vi "AM-Amplitude Modulation-Sound Output.vi"() -> ()   [LabVIEW 2016]
uses:
  <vilib>/sound2/lvsound2.llb/Sound Data Format.ctl
  <vilib>/Platform/TimedLoop/XDataNode/timing_clust.ctl
  <vilib>/Platform/TimedLoop/XDataNode/nitl_modes.ctl
  <vilib>/Platform/TimedLoop/XDataNode/wakeup.ctl
  <vilib>/measure/maspectr.llb/FFT Power Spectrum for 1 Chan.vi
  <vilib>/sound2/lvsound2.llb/Sound Output Write (DBL Single).vi
  <vilib>/Platform/TimedLoop/XDataNode/XDataNode.xnode
  <vilib>/Analysis/NI_AALBase.lvlib
  <vilib>/measure/NI_MAPro.lvlib
  <vilib>/Platform/TimedLoop/XDataNode/XDNodeRunTimeDep.lvlib
panel:
  in  "device ID":u32
  out "Data Signal":waveform(dbl)(graph) caption="Data Wave (Time Domain)"
  out "AM Modulated Signal (Frequency Domain)":cluster{"f0":dbl, "df":dbl, "magnitude":dbl[]}(graph) caption="AM Wave in Frequency Domain"
  out "Carrier Signal":waveform(dbl)(graph) caption="Carrier Wave (Time Domain)"
  out "AM Modulated Signal (Time Domain)":waveform(dbl)(graph) caption="AM Wave in Time Domain"
  in  "Carrier Amplitude":dbl(slide)=0.5 caption="Amplitude" min=0.0 max=1.0 scale=0.0..1.0
  in  "Data Frequency":dbl(slide)=40.0 caption="Frequency" scale=0.0..200.0
  in  "stop":bool
  in  "Data Amplitude":dbl(slide)=0.5 caption="Amplitude" min=0.0 max=1.0 scale=0.0..1.0
  in  "Carrier Frequency":dbl(slide)=400.0 caption="Frequency" scale=0.0..2000.0
  # "AM - Amplitude Modulation"
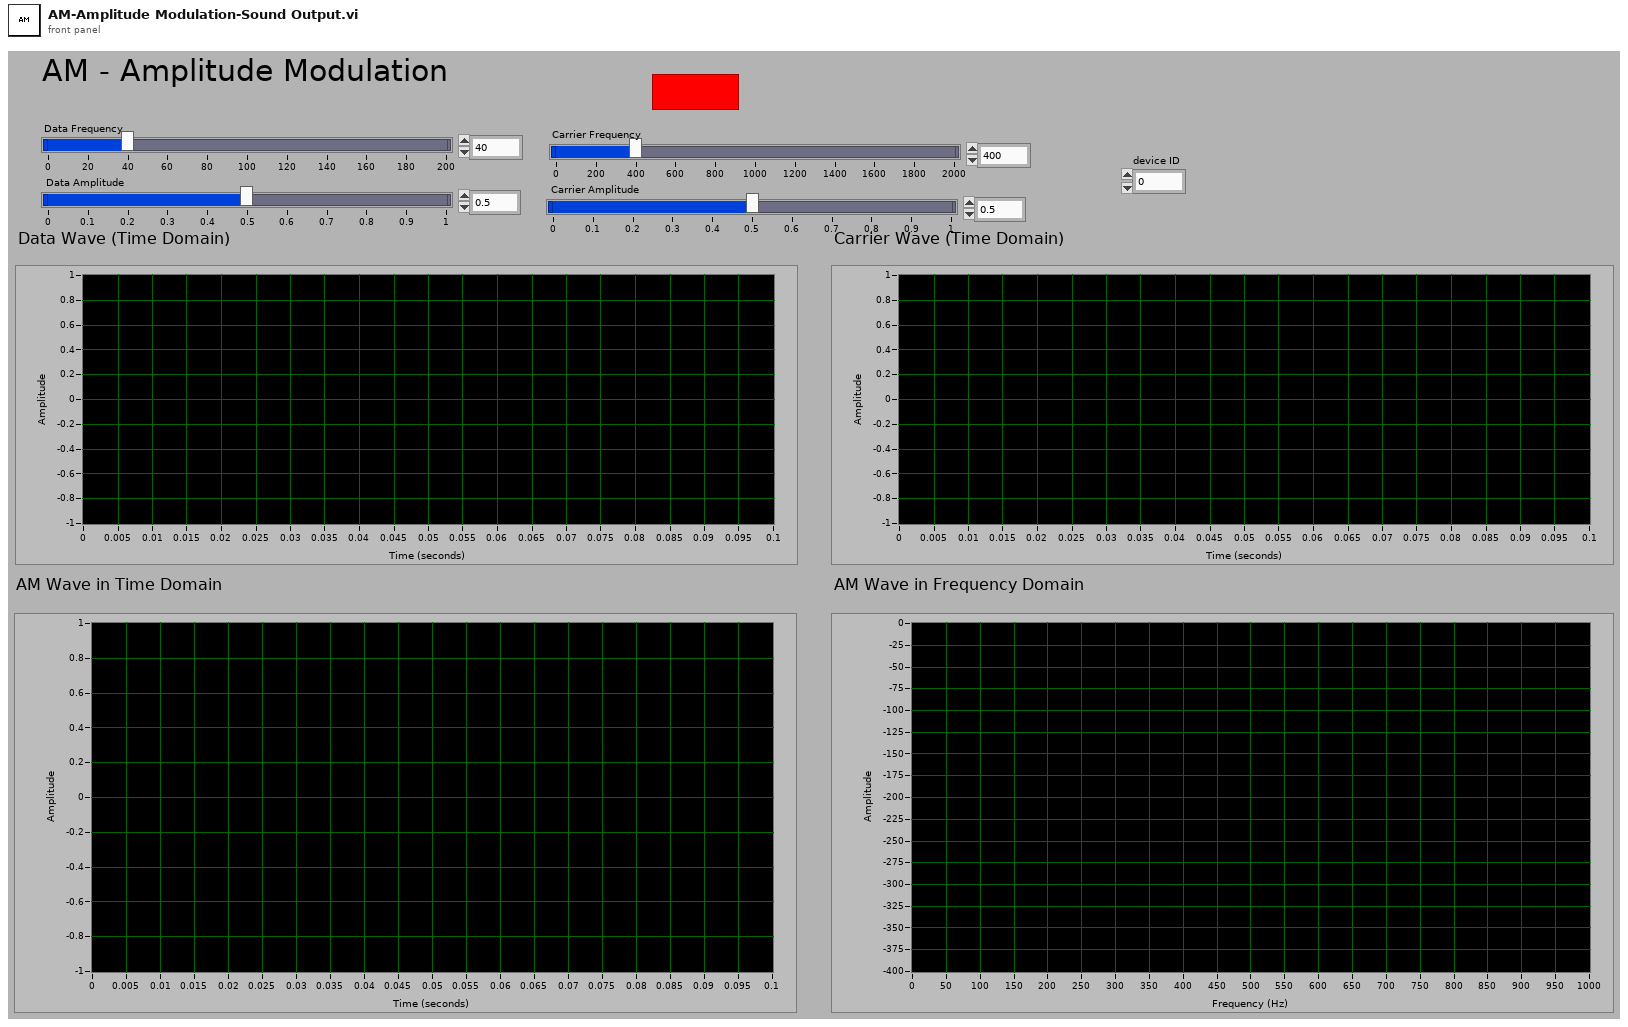
[diagram p1: front panel]
types:
  T1 = typedef "Sound Data Format.ctl" = cluster{"sample rate (S/s)":dbl, "number of channels":i32, "bits per sample":i32}
  T2 = typedef "Sound Output Task ID.ctl" = u32
  T3 = typedef "XDNodeRunTimeDep.lvlib/timing_clust.ctl" = cluster{"Expected End [f-1]":u64, "Actual End [f-1]":u64, "Finished Late? [f-1]":bool, "Expected End [i-1]":u64, "Actual End [i-1]":u64, "Finished Late? [i-1]":bool, "Expected Start [i]":u64, "Actual Start [i]":u64, "Expected Start [f]":u64, "Actual Start [f]":u64, "Source Name":string, "Structure Name":string, "Period":i64, "Deadline":i64, "Offset":i64, "Start":i64, "Priority":i32, "Timeout":i32, "Mode":T4, "Wakeup Reason":T5, "Error":errorcluster, "Source Type":string, "Secondary Source Type":string, "Global End Time":u64, "Global Start Time":u64, "Frame Duration":u64, "Iteration Duration":u64, "Assigned CPU":i32, "I/O Scan Engine Mode":u32}
  T4 = typedef "XDNodeRunTimeDep.lvlib/nitl_modes.ctl" = enum32{"No Change", "Process missed periods, maintain original phase", "Discard missed periods, maintain original phase", "Process missed periods, ignore original phase", "Discard missed periods, ignore original phase"}
  T5 = typedef "XDNodeRunTimeDep.lvlib/wakeup.ctl" = enum32{"Normal", "Aborted", "Asynchronous wakeup", "Timing source error", "Timed loop error", "Timeout"}
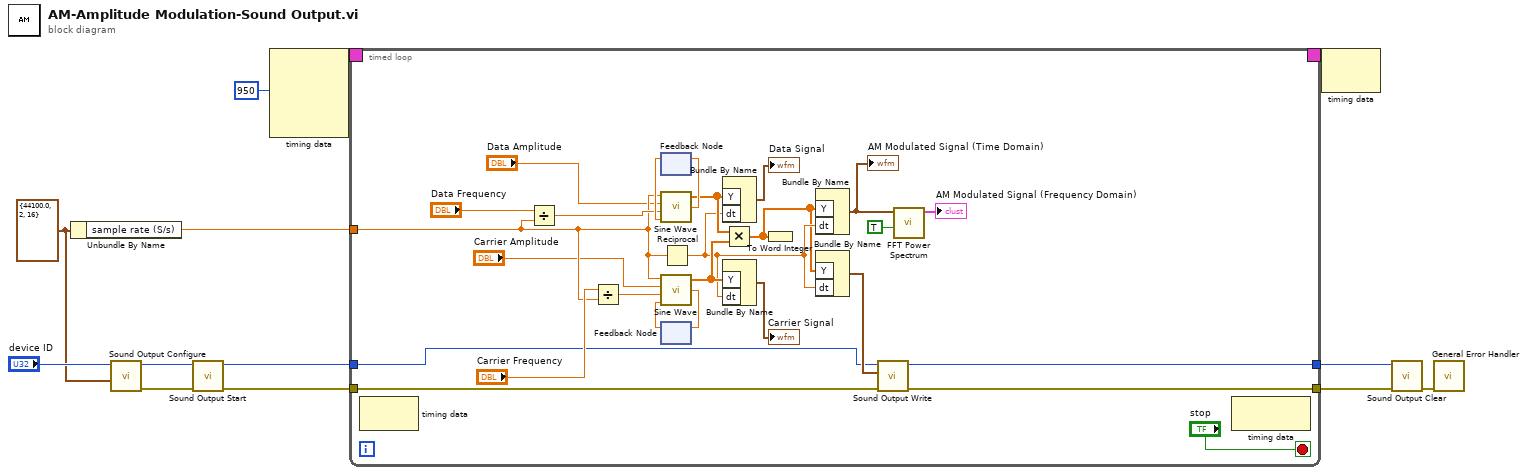
[diagram p0: block diagram]
diagram:
  w5 = T1 {"sample rate (S/s)"=44100.0, "number of channels"=2, "bits per sample"=16} ("sound format")
  n1 = Unbundle By Name(w5) -> ("sample rate (S/s)"=w4:dbl)
  n2 = call <vilib>:"Sound Output Configure.vi"("sound format"=w5, "device ID"="device ID") -> ("error out"=w11:errorcluster, "task ID"=w12:T2)  [unwired: 8 in]
  n3 = call <vilib>:"Sound Output Start.vi"("error in (no error)"=w11, "task ID"=w12) -> ("error out"=w9:errorcluster, "task ID out"=w10:T2)  [unwired: 8 in]
  n4 = node-c288(i64 950 ("Period")) -> (w3:T3)  [unwired: 3 in]
  n5 = timed-loop {
    tunnel: w10 -> [w18]
    tunnel: w9 -> [w17]
    tunnel: [w21] -> w8
    tunnel: [w20] -> w7
    tunnel: w4 -> [w30]
    timing: w3 -> [_]
    timing-out: [_] -> w2
    stop <- "stop" stop-if-true
    n6 = node-c288() -> ()  [unwired: 1 in, 1 out]
    n7 = Divide(x="Data Frequency", y=w30) -> (x/y=w35:dbl)
    n8 = Divide(x="Carrier Frequency", y=w30) -> (x/y=w31:dbl)
    n9 = feedback #1() -> (w37:dbl)  [unwired: 1 in]
    n10 = call <vilib>:"Sine Wave.vi"("samples"=w30, "amplitude"="Data Amplitude", "frequency"=w35, "phase in"=w37) -> ("sine wave"=w28:dbl[], "phase out"=w38:dbl)  [unwired: 1 in, 1 out]
    n11 = feedback-in #1(w38) -> ()
    n12 = feedback #2() -> (w34:dbl)  [unwired: 1 in]
    n13 = call <vilib>:"Sine Wave.vi"("samples"=w30, "amplitude"="Carrier Amplitude", "frequency"=w31, "phase in"=w34) -> ("sine wave"=w29:dbl[], "phase out"=w33:dbl)  [unwired: 1 in, 1 out]
    n14 = feedback-in #2(w33) -> ()
    n15 = Reciprocal(x=w30) -> (1/x=w19:dbl)
    n16 = Bundle By Name("Y"=w28, "dt"=w19) -> (→"Data Signal":waveform(dbl))  [unwired: 1 in]
    n17 = Bundle By Name("Y"=w29, "dt"=w19) -> (→"Carrier Signal":waveform(dbl))  [unwired: 1 in]
    n18 = Multiply(x=w28, y=w29) -> (x*y=w16:dbl[])
    n19 = To Word Integer(number=w16) -> ()  [unwired: 1 out]
    n20 = Bundle By Name("Y"=w16, "dt"=w19) -> (w25:waveform(dbl))  [unwired: 1 in]
    "AM Modulated Signal (Time Domain)" <- w25
    n21 = Bundle By Name("Y"=w16, "dt"=w19) -> (w22:waveform(dbl))  [unwired: 1 in]
    n22 = call-poly <vilib>:"Sound Output Write.vi"("error in (no error)"=w17, "data"=w22, "task ID"=w18) -> ("error out"=w20:errorcluster, "task ID out"=w21:T2)  [unwired: 7 in]
    n23 = call-poly <vilib>:"FFT Power Spectrum.vi"("dB On (F)"=TRUE, "time signal"=w25) -> ("power spectrum"=→"AM Modulated Signal (Frequency Domain)":cluster{"f0":dbl, "df":dbl, "magnitude":dbl[]})  [unwired: 6 in, 3 out]
    n24 = node-c288() -> ()  [unwired: 1 in, 1 out]
  }
  n25 = node-c288(w2) -> ()  [unwired: 1 out]
  n26 = call <vilib>:"Sound Output Clear.vi"("error in (no error)"=w7, "task ID"=w8) -> ("error out"=w6:errorcluster)  [unwired: 9 in]
  n27 = call <vilib>:"General Error Handler.vi"("error in (no error)"=w6) -> ()  [unwired: 2 in, 13 out]
